vi "Version.vi"() -> (2 "Version":string)   [LabVIEW 2017]
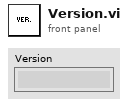
[diagram p1: front panel]
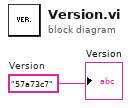
[diagram p0: block diagram]
diagram:
  w1 = "57a73c7"  # Version
  "Version" <- w1
